vi "ep_Y to D convert (Spectra).vi"(8 "error in (no error)":errorcluster, 11 "phase voltage spectra":T2(array[cluster])) -> (0 "error out":errorcluster, 3 "line voltage spectra":T2(array[cluster]))   [LabVIEW 2014, in "NI_EP_Power Quality.lvlib"]
uses:
  <vilib>/addons/Electrical Power/PQ/NI_EP_Power Quality.lvlib
  <vilib>/addons/Electrical Power/PQ/Common/Controls/ep_AI Data Channel.ctl
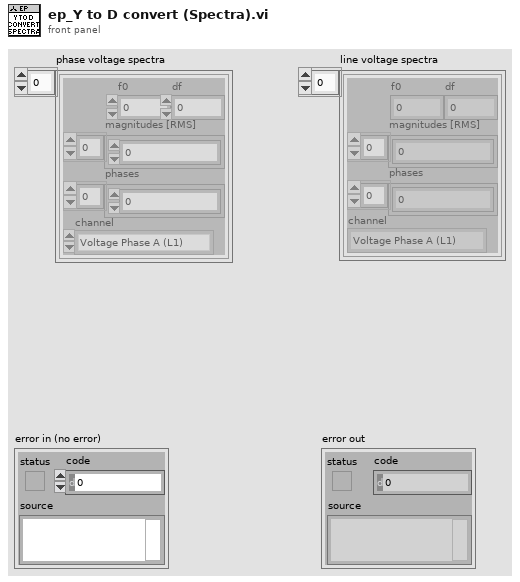
[diagram p1: front panel]
types:
  T1 = typedef "NI_EP_Power Quality.lvlib/ep_AI Data Channel.ctl" = enum16{"Voltage Phase A (L1)", "Voltage Phase B (L2)", "Voltage Phase C (L3)", "Voltage Phase N (Neutral)", "Current Phase A (L1)", "Current Phase B (L2)", "Current Phase C (L3)", "Current Phase N (Neutral)"}
  T2 = cluster{"f0":dbl, "df":dbl, "magnitudes [RMS]":dbl[], "phases":dbl[], "channel":T1}[]
  T3 = cluster{"f0":dbl, "df":dbl, "magnitudes [RMS]":dbl[], "phases":dbl[], "channel":T1}
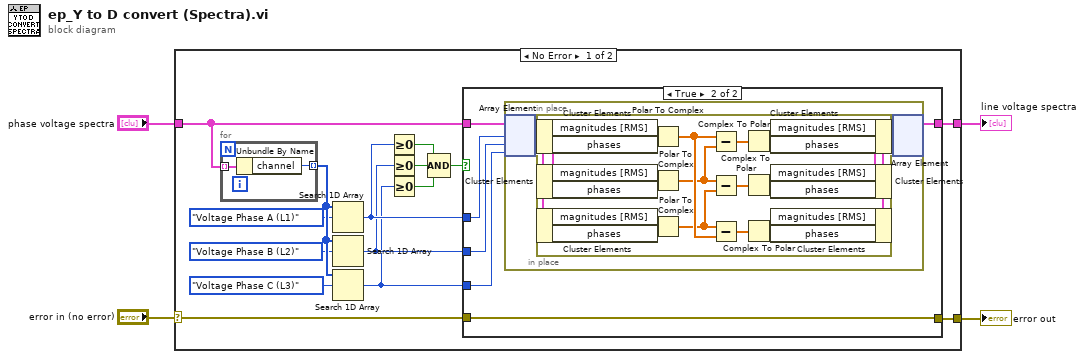
[diagram p0: block diagram]
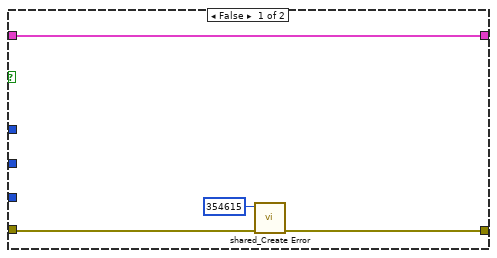
[diagram p2: hidden frame]
diagram:
  n1 = case shown="No Error" "error in (no error)" {
    selector: "error in (no error)" -> [w6 w56]
    tunnel: "phase voltage spectra" -> [w19 _]
    tunnel: [w18 _] -> w2
    tunnel: [w5 w56] -> w1
    frame No Error {
      n2 = for {
        tunnel: w19 -> [w21] mode=indexing
        tunnel: [w20] -> w15 mode=indexing
        n3 = Unbundle By Name(w21) -> ("channel"=w20:T1)
      }
      n4 = Search 1D Array(1D array=w15, element=ep_AI_Data_Channel."Voltage Phase A (L1)" ("AI data channel")) -> (index of element=w10:i32)  [unwired: 1 in]
      n5 = Search 1D Array(1D array=w15, element=ep_AI_Data_Channel."Voltage Phase B (L2)" ("AI data channel")) -> (index of element=w8:i32)  [unwired: 1 in]
      n6 = Search 1D Array(1D array=w15, element=ep_AI_Data_Channel."Voltage Phase C (L3)" ("AI data channel")) -> (index of element=w7:i32)  [unwired: 1 in]
      n7 = Greater Or Equal To 0?(x=w10) -> (x >= 0?=w11:bool)
      n8 = Greater Or Equal To 0?(x=w8) -> (x >= 0?=w16:bool)
      n9 = Greater Or Equal To 0?(x=w7) -> (x >= 0?=w17:bool)
      n10 = Compound Arithmetic op=AND(w11, w16, w17) -> (w9:bool)
      n11 = case shown="True" w9 {
        tunnel: [w25 w30] -> w18
        tunnel: w19 -> [w25 w31]
        tunnel: w10 -> [_ w29]
        tunnel: w8 -> [_ w28]
        tunnel: w7 -> [_ w27]
        tunnel: w6 -> [w23 w26]
        tunnel: [w22 w26] -> w5
        frame False {
          n12 = call <vilib>:"shared_Create Error.vi"("error in (no error)"=w23, "error code (0)"=354615) -> ("error out"=w22:errorcluster)  [unwired: 9 in]
        }
        frame True {
          n13 = in-place {
            n14 = in-place-array #1(w31, w29, w28, w27) -> (w37:T3, w36:T3, w35:T3)
            n15 = in-place {
              n16 = in-place-cluster #2(w37) -> ("magnitudes [RMS]"=w54:dbl[], "phases"=w55:dbl[])
              n17 = in-place-cluster #3(w36) -> ("magnitudes [RMS]"=w49:dbl[], "phases"=w48:dbl[])
              n18 = in-place-cluster #4(w35) -> ("magnitudes [RMS]"=w45:dbl[], "phases"=w46:dbl[])
              n19 = Polar To Complex(1:w55, 2:w54) -> (0:w53:cdb[])
              n20 = Polar To Complex(1:w48, 2:w49) -> (0:w47:cdb[])
              n21 = Polar To Complex(1:w46, 2:w45) -> (0:w44:cdb[])
              n22 = Subtract(x=w53, y=w47) -> (x-y=w52:cdb[])
              n23 = Subtract(x=w47, y=w44) -> (x-y=w42:cdb[])
              n24 = Subtract(x=w44, y=w53) -> (x-y=w43:cdb[])
              n25 = Complex To Polar(r * e^(i*theta)=w52) -> (r=w51:dbl[], theta=w50:dbl[])
              n26 = Complex To Polar(r * e^(i*theta)=w42) -> (r=w41:dbl[], theta=w40:dbl[])
              n27 = Complex To Polar(r * e^(i*theta)=w43) -> (r=w39:dbl[], theta=w38:dbl[])
              n28 = in-place-cluster #2("magnitudes [RMS]"=w51, "phases"=w50) -> (w34:T3)
              n29 = in-place-cluster #3("magnitudes [RMS]"=w41, "phases"=w40) -> (w33:T3)
              n30 = in-place-cluster #4("magnitudes [RMS]"=w39, "phases"=w38) -> (w32:T3)
            }
            n31 = in-place-array #1(w34, w33, w32) -> (w30:T2)  [unwired: 3 out]
          }
        }
      }
    }
    frame Error {
    }
  }
  "error out" <- w1
  "line voltage spectra" <- w2
